vi "Set Group by Date.vi"(8 "error in (no error)":errorcluster, 10 "Group by Date?":bool, 11 "Report Generator In":refnum<class "Report Generator.lvclass">) -> (0 "error out":errorcluster, 3 "Report Generator Out":refnum<class "Report Generator.lvclass">)   [LabVIEW 2020, in "Report Generator.lvclass"]
uses:
  Report Generator.lvclass
  C:/Git/astemes-lunit/source/Application Framework/Process Classes/Process/Process.lvclass
  Application Framework/Process Classes/Process/Process.lvclass/Process.ctl
  Application Framework/Process Classes/Process/Process.lvclass
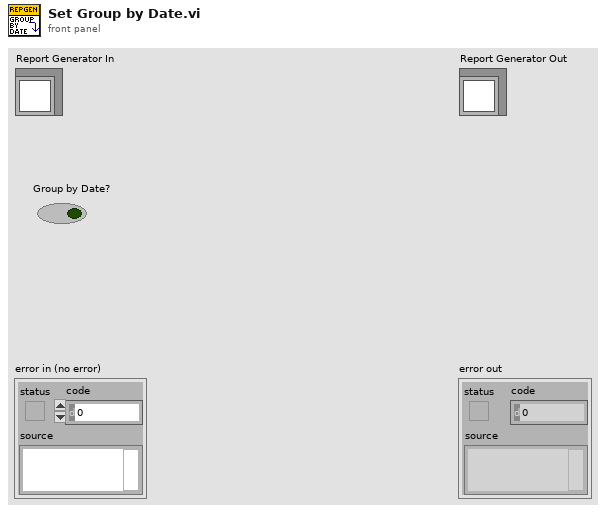
[diagram p1: front panel]
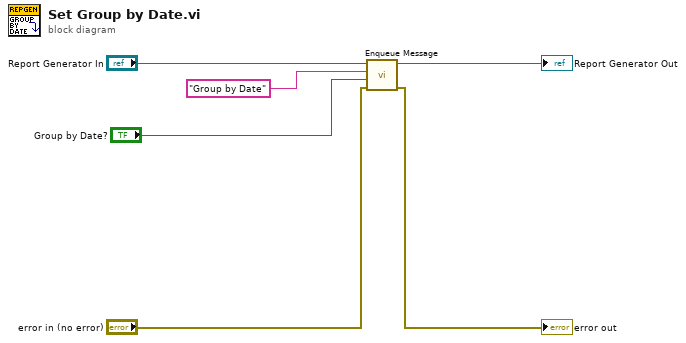
[diagram p0: block diagram]
diagram:
  n1 = call "Enqueue Message.vi"("error in (no error)"="error in (no error)", "Message Data"="Group by Date?", "Message"="Group by Date", "Process In"="Report Generator In") -> ("error out"=→"error out":errorcluster, "Process Out"=→"Report Generator Out":refnum<class "Report Generator.lvclass">)  [unwired: 6 in]
